vi "Read Device Signals.vi"(8 "error in":errorcluster, 11 "Config in":refnum<class "Config.lvclass">) -> (0 "error out":errorcluster, 2 "Device_Signals":string[][](array[string]), 3 "Config out":refnum<class "Config.lvclass">)   [LabVIEW 2023, in "Config.lvlib" / "Config.lvclass"]
uses:
  Config.lvclass
  Config.lvclass/Config.ctl
  builds/Tools/SLL.lvlibp/Accessors/Read Device Data.vi
  builds/Tools/SLL.lvlibp/SLL.lvclass
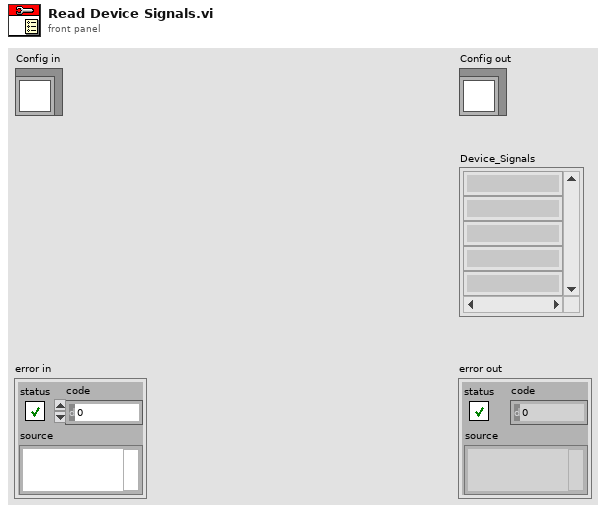
[diagram p1: front panel]
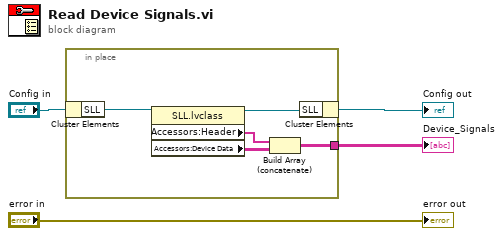
[diagram p0: block diagram]
diagram:
  n1 = in-place {
    in-place-border: [w5] -> w2
    n2 = in-place-cluster #1("Config in") -> ("SLL"=w9:refnum<class "SLL.lvclass">)
    n3 = property class="SLL.lvclass"(reference=w9) -> (reference out=w8:refnum<class "SLL.lvclass">, "Accessors:Header"=w7:string[], "Accessors:Device Data"=w6:string[][])  [unwired: 1 in, 1 out]
    n4 = Build Array (concatenate)(w7, w6) -> (w5:string[][])
    n5 = in-place-cluster #1("SLL"=w8) -> (→"Config out":refnum<class "Config.lvclass">)
  }
  "Device_Signals" <- w2
  "error out" <- "error in"
